vi "Flom pump Control 11-30.vi"() -> ()   [LabVIEW 2009]
doc: "Use this template to parse data you acquired from an instrument and write the data to a file.\nNote: LabVIEW enables automatic error handling by default for VIs you create from this template."
panel:
  in  "stop 2":bool
  out "Output":string
  in  "Execute Button":bool
  in  "Step Flow Commands \n(Only For Step Flow)":string(combo)
  in  "Time (.01 mins)":i32 min=0 max=9999 step=1
  in  "Step #":i32=1 min=0 max=49 step=1
  in  "Stop   Start":bool=TRUE
  in  "Flow Rate (uL)":i32 min=0 max=9900 step=1
  in  "Edit Values, or Run Flow?\n(Only for Continuous Flow)":string(combo)
  in  "Setup Commands\n(Only for Setup)":string(combo)
  in  "Mode":string(combo)="Setup"
  in  "Request Commands\n(Only for Status)":string(combo)
  in  "Pump #?":i32 min=1 max=2 step=1
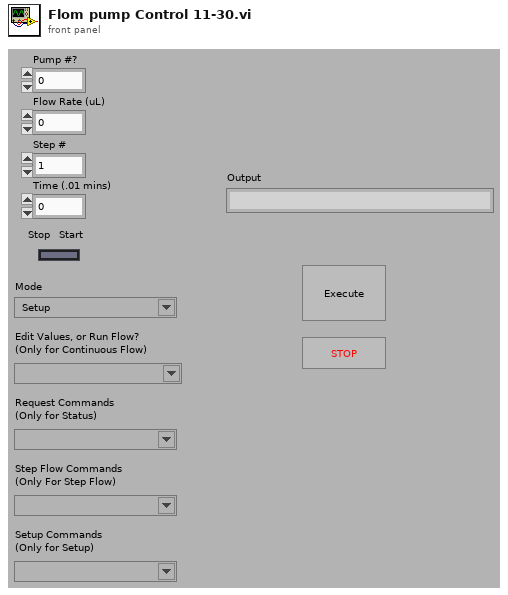
[diagram p1: front panel]
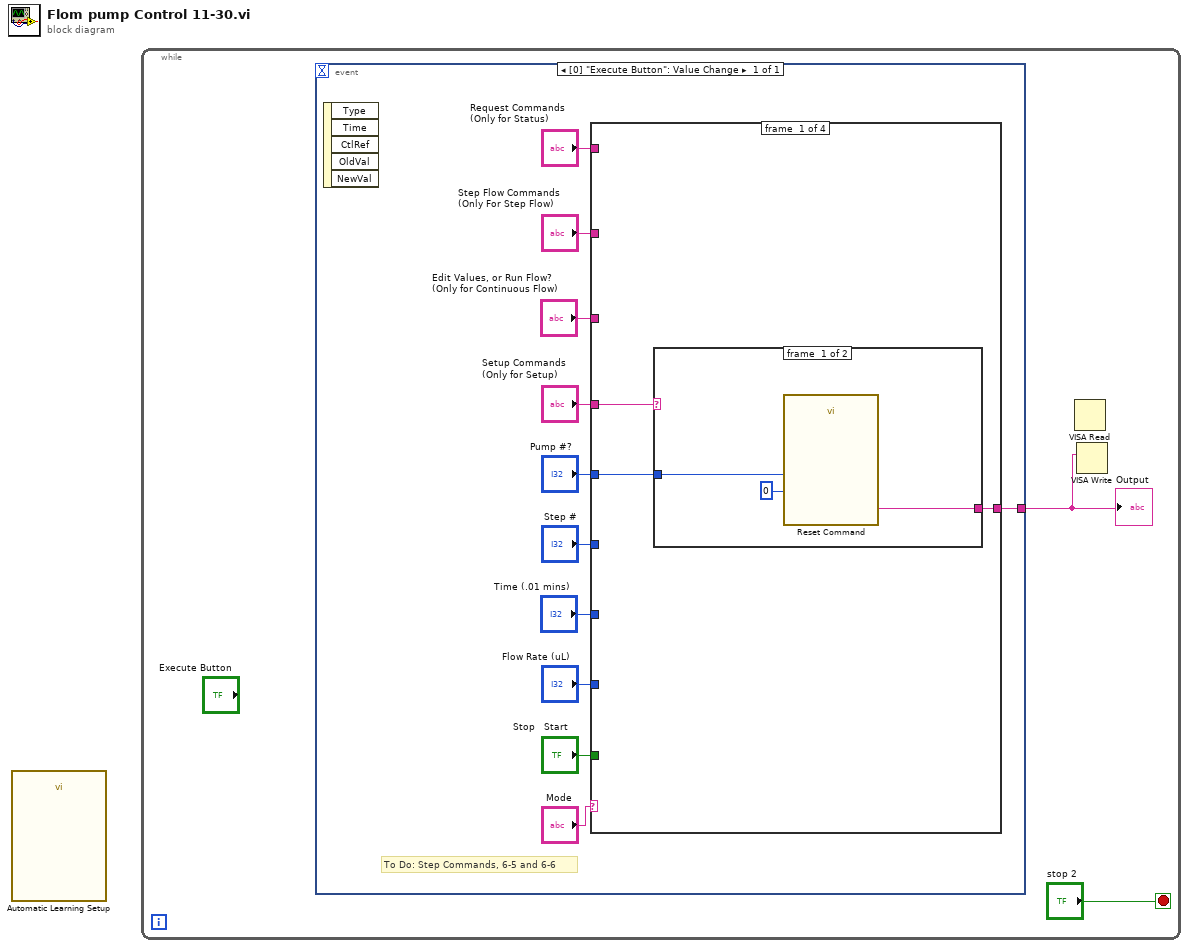
[diagram p0: block diagram]
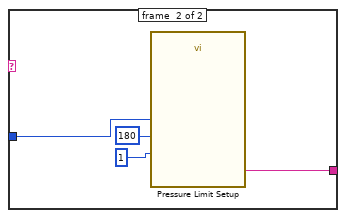
[diagram p2: hidden frame]
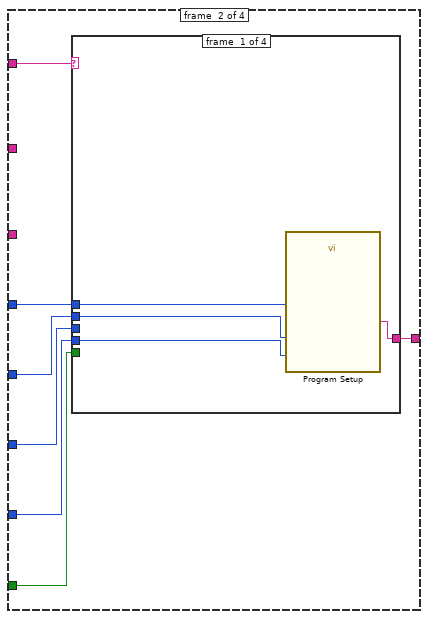
[diagram p3: hidden frame]
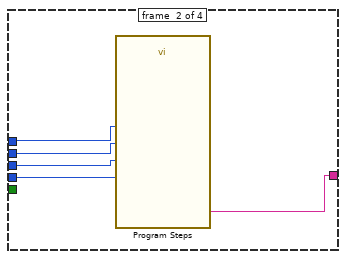
[diagram p4: hidden frame]
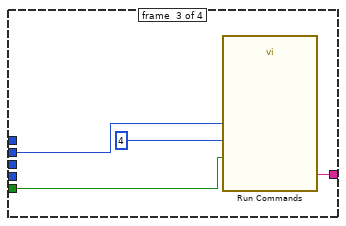
[diagram p5: hidden frame]
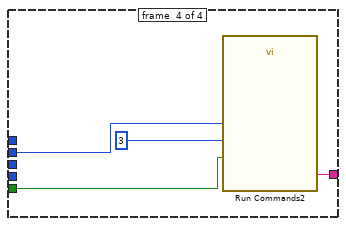
[diagram p6: hidden frame]
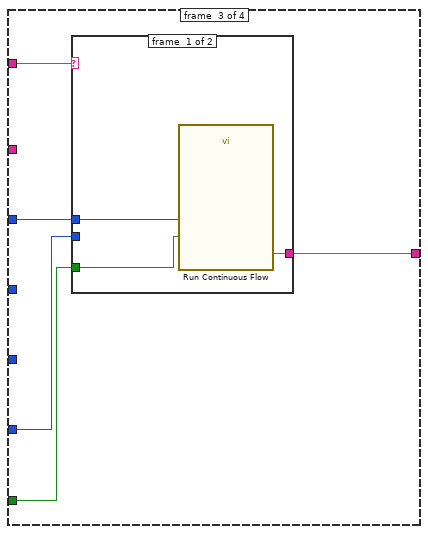
[diagram p7: hidden frame]
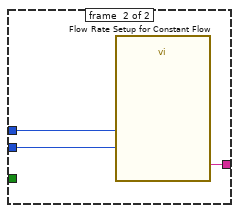
[diagram p8: hidden frame]
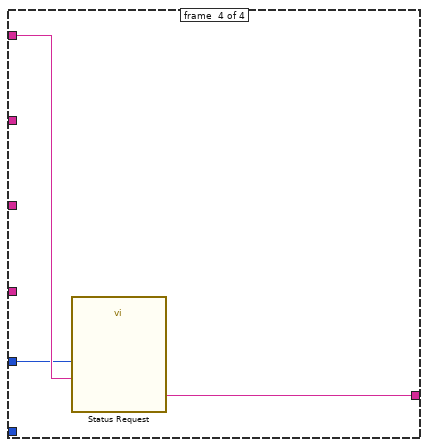
[diagram p9: hidden frame]
diagram:
  n1 = call "Automatic Learning Setup"() -> ()  [unwired: 4 in, 12 out]
  n2 = while {
    stop <- "stop 2" stop-if-true
    n3 = event shown="[0] \"Execute Button\": Value Change" {
      selector: _ -> [_]
      dyn-events: _ -> [_]
      timeout: _ -> [_]
      tunnel: [w3] -> w1
      event [0] "Execute Button": Value Change {
        # "To Do: Step Commands, 6-5 and 6-6"
        n4 = event-data() -> ()  [unwired: 6 out]
        n5 = case shown="\"Step Flow\"" "Mode" {
          tunnel: "Pump #?" -> [w15 w30 w52 w60]
          tunnel: "Request Commands\n(Only for Status)" -> [_ _ _ w61]
          tunnel: "Setup Commands\n(Only for Setup)" -> [w16 _ _ _]
          tunnel: "Edit Values, or Run Flow?\n(Only for Continuous Flow)" -> [_ _ w51 _]
          tunnel: "Flow Rate (uL)" -> [_ w27 w50 _]
          tunnel: "Stop   Start" -> [_ w24 w49 _]
          tunnel: [w14 w29 w48 w59] -> w3
          tunnel: "Step #" -> [_ w28 _ _]
          tunnel: "Time (.01 mins)" -> [_ w26 _ _]
          tunnel: "Step Flow Commands \n(Only For Step Flow)" -> [_ w25 _ _]
          frame #0 {
            n6 = case shown="\"Reset\", Default" w16 {
              tunnel: w15 -> [w19 w21]
              tunnel: [w17 w20] -> w14
              frame #0 {
                n7 = call "Reset Command"("pump"=w19, "reset command"=0) -> ("Result"=w17:string)  [unwired: 2 in, 11 out]
              }
              frame #1 {
                n8 = call "Pressure Limit Setup"("pump"=w21, "U Lim (0.1MPa)"=180, "L Lim (0.1MPa)"=1) -> ("Result"=w20:string)  [unwired: 2 in, 10 out]
              }
            }
          }
          frame #1 {
            n9 = case shown="\"Step Flow Rates\"" w25 {
              tunnel: w30 -> [w34 w38 _ _]
              tunnel: [w33 w35 w40 w47] -> w29
              tunnel: w28 -> [w32 w39 w43 w45]
              tunnel: w27 -> [w31 w37 _ _]
              tunnel: w26 -> [_ w36 _ _]
              tunnel: w24 -> [_ _ w42 w46]
              frame #0 {
                n10 = call "Program Setup"("pump"=w34, "Number of Steps"=w32, "Stepped Initial Flow Rate"=w31) -> ("Result"=w33:string)  [unwired: 2 in, 10 out]
              }
              frame #1 {
                n11 = call "Program Steps"("flow rate"=w37, "pump"=w38, "step number"=w39, "time .01 mins"=w36) -> ("Result"=w35:string)  [unwired: 3 in, 8 out]
              }
              frame #2 {
                n12 = call "Run Commands"("pump"=w43, "Flow mode"=4, "Start/Stop"=w42) -> ("Result"=w40:string)  [unwired: 2 in, 10 out]
              }
              frame #3 {
                n13 = call "Run Commands2"("pump"=w45, "Flow mode"=3, "Start/Stop"=w46) -> ("Result"=w47:string)  [unwired: 2 in, 10 out]
              }
            }
          }
          frame #2 {
            n14 = case shown="\"Edit\", Default" w51 {
              tunnel: w52 -> [w54 w58]
              tunnel: w50 -> [_ w57]
              tunnel: w49 -> [w55 _]
              tunnel: [w53 w56] -> w48
              frame #0 {
                n15 = call "Run Continuous Flow"("pump"=w54, "Start/Stop"=w55) -> ("Result"=w53:string)  [unwired: 2 in, 11 out]
              }
              frame #1 {
                n16 = call "Flow Rate Setup for Constant Flow"("pump"=w58, "flow rate in uL"=w57) -> ("Result"=w56:string)  [unwired: 2 in, 11 out]
              }
            }
          }
          frame #3 {
            n17 = call "Status Request"("pump"=w60, "query"=w61) -> ("Result"=w59:string)  [unwired: 2 in, 11 out]
          }
        }
      }
    }
    "Output" <- w1
    n18 = VISA Read() -> ()  [unwired: 3 in, 4 out]
    n19 = VISA Write(write buffer=w1) -> ()  [unwired: 2 in, 3 out]
  }
